vi "Parse Variable Container.vi"(6 "Parent Type":T2, 7 "Blacklist":string[](array[string]), 8 "error in (no error)":errorcluster, 9 "Top Level Folders in":T1[](array[typedef]), 10 "Variable Object":refnum<k21>, 11 "Tag Array In":refnum<class "Synchronised Tag.lvclass">[](array[class])) -> (0 "Error Out":errorcluster, 1 "Top Level Folders Out":T1[](array[typedef]), 3 "Tag Array Out":refnum<class "Synchronised Tag.lvclass">[](array[class]))   [LabVIEW 2016]
doc: "Takes a variable container as an input and recursively parses it for different OPC UA items."
uses:
  Controls/Node Type.ctl
  Sync Tag Class/Synchronised Tag.lvclass
  Controls/Folders to Add.ctl
  <resource>/objmgr/ni.var.rc
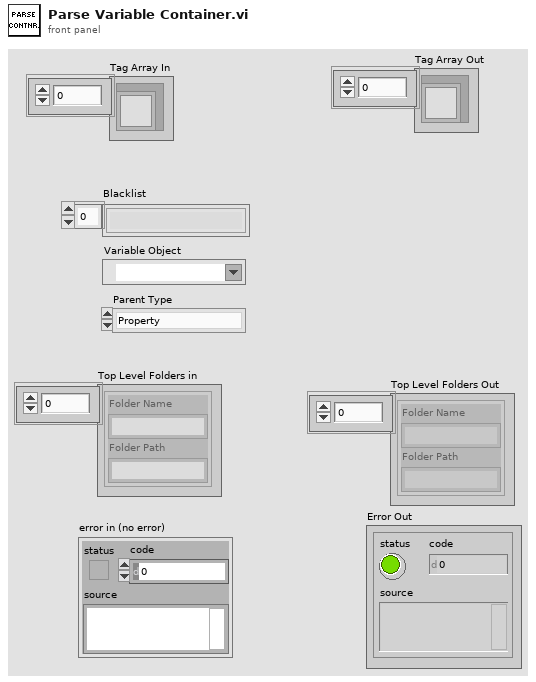
[diagram p1: front panel]
types:
  T1 = typedef "Folders to Add.ctl" = cluster{"Folder Name":string, "Folder Path":string}
  T2 = typedef "Node Type.ctl" = enum16{"Property", "Item", "Folder"}
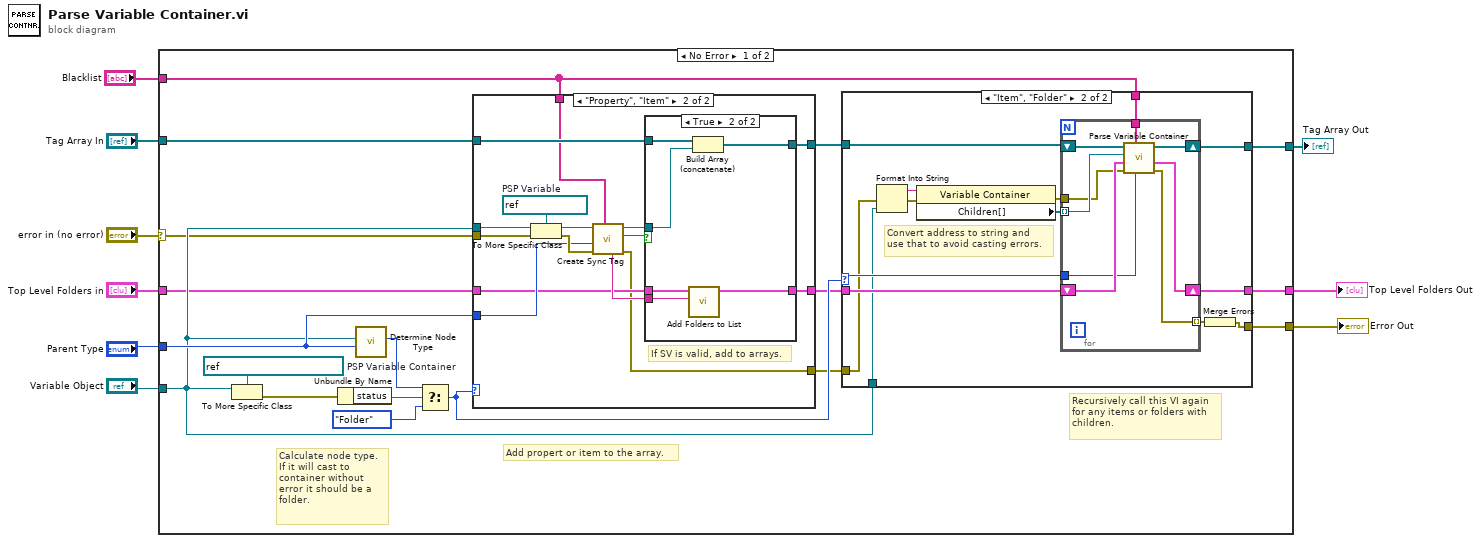
[diagram p0: block diagram]
diagram:
  n1 = case shown="No Error" "error in (no error)" {
    selector: "error in (no error)" -> [w11 w81]
    tunnel: "Parent Type" -> [w21 _]
    tunnel: "Tag Array In" -> [w20 w82]
    tunnel: [w17 w82] -> w1
    tunnel: "Blacklist" -> [w16 _]
    tunnel: [w15 w80] -> w6
    tunnel: [w13 w81] -> w5
    tunnel: "Variable Object" -> [w12 _]
    tunnel: "Top Level Folders in" -> [w10 w80]
    frame No Error {
      w27 = refnum<k21> refnum  # PSP Variable Container
      # "Add propert or item to the array."
      # "Recursively call this VI again\nfor any items or folders with\nchildren."
      # "Calculate node type.\nIf it will cast to \ncontainer without\nerror it should be a\nfolder."
      n2 = To More Specific Class(target class=w27, reference=w12) -> (error out=w26:errorcluster)  [unwired: 1 in, 1 out]
      n3 = Unbundle By Name(w26) -> ("status"=w25:bool)
      n4 = call "Determine Node Type.vi"("Parent Type"=w21, "Refnum in"=w12) -> ("Node Type"=w23:T2)  [unwired: 9 in]
      n5 = Select(t=w23, s=w25, f=Node_Type."Folder" ("Node Type")) -> (s? t:f=w22:T2)
      n6 = case shown="\"Property\", \"Item\"" w22 {
        tunnel: w12 -> [_ w70]
        tunnel: w21 -> [_ w67]
        tunnel: w20 -> [w56 w66]
        tunnel: [w56 w65] -> w19
        tunnel: w10 -> [w55 w62]
        tunnel: [w55 w61] -> w18
        tunnel: w16 -> [_ w60]
        tunnel: [w54 w59] -> w14
        tunnel: w11 -> [w54 w58]
        frame Default {
        }
        frame "Property", "Item" {
          w71 = refnum<k21> refnum  # PSP Variable
          # "If SV is valid, add to arrays."
          n7 = To More Specific Class(target class=w71, reference=w70, error in=w58) -> (specific class reference=w69:refnum<k21>, error out=w68:errorcluster)
          n8 = call "Create Sync Tag.vi"("Blacklist"=w60, "error in (no error)"=w68, "Parent Type"=w67, "Variable"=w69) -> ("error out"=w59:errorcluster, "Created?"=w63:bool, "Synchronised Tag"=w57:refnum<class "Synchronised Tag.lvclass">, "Folder"=w64:string)  [unwired: 4 in]
          n9 = case shown="True" w63 {
            tunnel: w66 -> [w72 w79]
            tunnel: w57 -> [_ w78]
            tunnel: [w72 w77] -> w65
            tunnel: w64 -> [_ w76]
            tunnel: w62 -> [w73 w74]
            tunnel: [w73 w75] -> w61
            frame False {
            }
            frame True {
              n10 = call "Add Folders to List.vi"("Folder"=w76, "Top Level Folders in"=w74) -> ("Top Level Folders Out"=w75:T1[])  [unwired: 9 in]
              n11 = Build Array (concatenate)(w79, w78) -> (w77:refnum<class "Synchronised Tag.lvclass">[])
            }
          }
        }
      }
      n12 = case shown="\"Item\", \"Folder\"" w22 {
        selector: w22 -> [_ w41]
        tunnel: w19 -> [w30 w44]
        tunnel: w18 -> [w29 w42]
        tunnel: [w30 w43] -> w17
        tunnel: [w29 w40] -> w15
        tunnel: w16 -> [_ w38]
        tunnel: w14 -> [w28 w34]
        tunnel: [w28 w37] -> w13
        tunnel: w12 -> [_ w31]
        frame Default {
        }
        frame "Item", "Folder" {
          # "Convert address to string and \nuse that to avoid casting errors."
          n13 = Format Into String(error in=w34, w31) -> (resulting string=w36:string, error out=w35:errorcluster)  [unwired: 2 in]
          n14 = property class="Variable Container"(reference=w36, error in=w35) -> (error out=w32:errorcluster, "Children[]"=w39:refnum<k21>[])  [unwired: 1 out]
          n15 = for {
            shift-right: [w52] -> w43
            shift-left: w44 -> [w53]
            tunnel: w41 -> [w50]
            shift-right: [w49] -> w40
            shift-left: w42 -> [w51]
            tunnel: w39 -> [w48] mode=indexing
            tunnel: w38 -> [w47]
            tunnel: [w45] -> w33 mode=indexing
            tunnel: w32 -> [w46]
            n16 = call "Parse Variable Container.vi"("Parent Type"=w50, "Blacklist"=w47, "error in (no error)"=w46, "Top Level Folders in"=w51, "Variable Object"=w48, "Tag Array In"=w53) -> ("Error Out"=w45:errorcluster, "Top Level Folders Out"=w49:T1[], "Tag Array Out"=w52:refnum<class "Synchronised Tag.lvclass">[])  [unwired: 3 in]
          }
          n17 = Merge Errors(w33) -> (w37:errorcluster)
        }
      }
    }
    frame Error {
    }
  }
  "Top Level Folders Out" <- w6
  "Error Out" <- w5
  "Tag Array Out" <- w1
